vi "CMD_PRINT.vi"(6 "Gantry in":refnum<class "Gantry.lvclass">, 7 "Console Log in":refnum<class "Console Log.lvclass">, 8 "error in (no error)":errorcluster, 9 "Timestamp":bool=TRUE, 10 "Arguments":string[](array[string]), 11 "gScript Interpreter in":refnum<class "gScript Interpreter.lvclass">) -> (0 "error out":errorcluster, 3 "gScript Interpreter out":refnum<class "gScript Interpreter.lvclass">, 4 "Gantry out":refnum<class "Gantry.lvclass">, 5 "Console Log out":refnum<class "Console Log.lvclass">)   [LabVIEW 2026, in "gScript Interpreter.lvclass"]
uses:
  gScript Interpreter.lvclass
  Application Utilities/Console Log/Console Log.lvclass
  Shared Components/Gantry Class/Gantry.lvclass
  <vilib>/regexp/Match Regular Expression.xnode
  gScript Interpreter.lvclass/gScript Interpreter.ctl
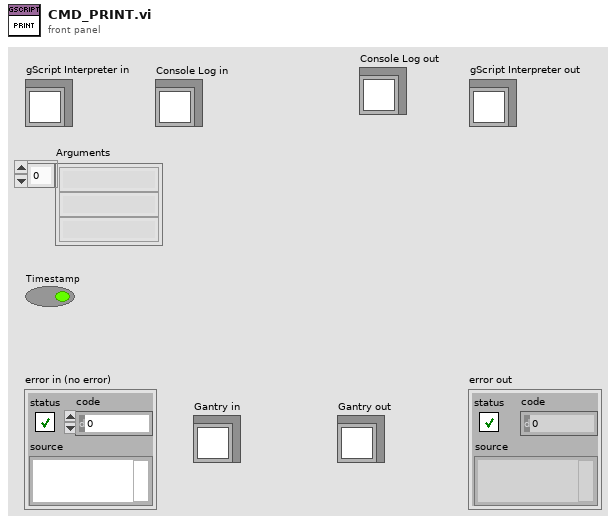
[diagram p1: front panel]
types:
  T1 = typedef "Memory Cell.ctl" = cluster{"type":T2, "x":dbl, "y":dbl, "z":dbl, "w":dbl}
  T2 = typedef "Memory Cell Type Enum.ctl" = enum16{"integer", "float", "vector", "rotation"}
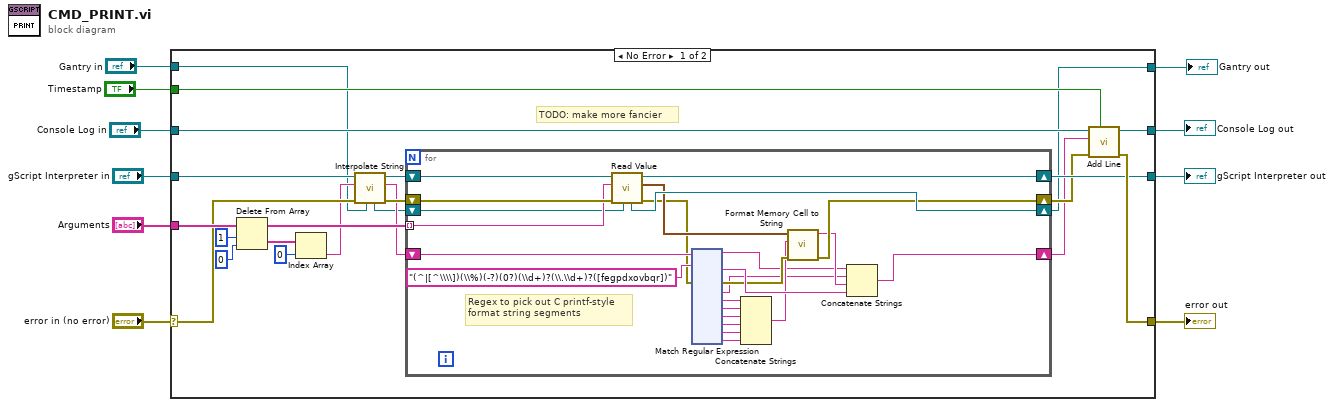
[diagram p0: block diagram]
diagram:
  n1 = case shown="No Error" "error in (no error)" {
    selector: "error in (no error)" -> [w18 w185]
    tunnel: [w30 w185] -> w9
    tunnel: [w23 w184] -> w7
    tunnel: "gScript Interpreter in" -> [w19 w184]
    tunnel: "Arguments" -> [w29 _]
    tunnel: "Console Log in" -> [w32 w183]
    tunnel: [w31 w183] -> w4
    tunnel: "Timestamp" -> [w20 _]
    tunnel: "Gantry in" -> [w13 w182]
    tunnel: [w11 w182] -> w1
    frame No Error {
      # "TODO: make more fancier"
      n2 = Delete From Array(array=w29, length=1, index=0) -> (deleted portion=w25:string[], array with subset deleted=w28:string[])
      n3 = Index Array(array=w25, index=0) -> (element=w15:string)
      n4 = call-dynamic "Interpolate String.vi"("Gantry in"=w13, "error in (no error)"=w18, "Input String"=w15, "gScript Interpreter in"=w19) -> ("error out"=w17:errorcluster, "Output String"=w14:string, "gScript Interpreter out"=w16:refnum<class "gScript Interpreter.lvclass">, "Gantry out"=w12:refnum<class "Gantry.lvclass">)  [unwired: 4 in]
      n5 = for {
        tunnel: w28 -> [w54] mode=indexing
        shift-right: [w53] -> w23
        shift-left: w16 -> [w56]
        shift-right: [w47] -> w22
        shift-left: w17 -> [w55]
        shift-right: [w42] -> w21
        shift-left: w14 -> [w50]
        shift-right: [w51] -> w11
        shift-left: w12 -> [w52]
        # "Regex to pick out C printf-style\nformat string segments"
        n6 = call-dynamic "Read Value.vi"("Gantry in"=w52, "error in (no error)"=w55, "String in"=w54, "gScript Interpreter in"=w56) -> ("error out"=w44:errorcluster, "Memory Cell"=w48:T1, "gScript Interpreter out"=w53:refnum<class "gScript Interpreter.lvclass">, "Gantry out"=w51:refnum<class "Gantry.lvclass">)  [unwired: 4 in]
        n7 = xnode "Match Regular Expression"("input string"=w50, "regular expression"="(^|[^\\\\])(\\%)(-?)(0?)(\\d+)?(\\.\\d+)?([fegpdxovbqr])", "error in"=w44) -> ("before match"=w34:string, "after match"=w45:string, "error out"=w43:errorcluster, "submatch 1"=w33:string, "submatch 2"=w41:string, "submatch 3"=w40:string, "submatch 4"=w39:string, "submatch 5"=w38:string, "submatch 6"=w36:string, "submatch 7"=w35:string)  [unwired: 3 in, 2 out]
        n8 = Concatenate Strings(w41, w40, w39, w38, w36, w35) -> (w37:string)
        n9 = call "Format Memory Cell to String.vi"("error in (no error)"=w43, "Format String"=w37, "Memory Cell"=w48) -> ("error out"=w47:errorcluster, "output string"=w46:string)  [unwired: 7 in]
        n10 = Concatenate Strings(w34, w33, w46, w45) -> (w42:string)
      }
      n11 = call "Add Line.vi"("Timestamp"=w20, "error in"=w22, "String"=w21, "Console Log in"=w32) -> ("error out"=w30:errorcluster, "Console Log out"=w31:refnum<class "Console Log.lvclass">)  [unwired: 6 in]
    }
    frame Error {
    }
  }
  "error out" <- w9
  "gScript Interpreter out" <- w7
  "Console Log out" <- w4
  "Gantry out" <- w1
